vi "Write Page Properties.vi"(8 "error in (no error)":errorcluster, 10 "Page Properties":T1[](array[typedef]), 11 "CustomDeviceRepo in":refnum<class "CustomDeviceRepo.lvclass">) -> (0 "error out":errorcluster, 3 "CustomDeviceRepo out":refnum<class "CustomDeviceRepo.lvclass">)   [LabVIEW 2014, in "CustomDeviceRepo.lvclass"]
uses:
  CustomDeviceRepo.lvclass
  Custom Device Type Defs/Page Properties.ctl
  Custom Device XML/Custom Device XML/Path Cluster.ctl
  Custom Device XML/Custom Device XML/help.ctl
  CustomDeviceRepo.lvclass/CustomDeviceRepo.ctl
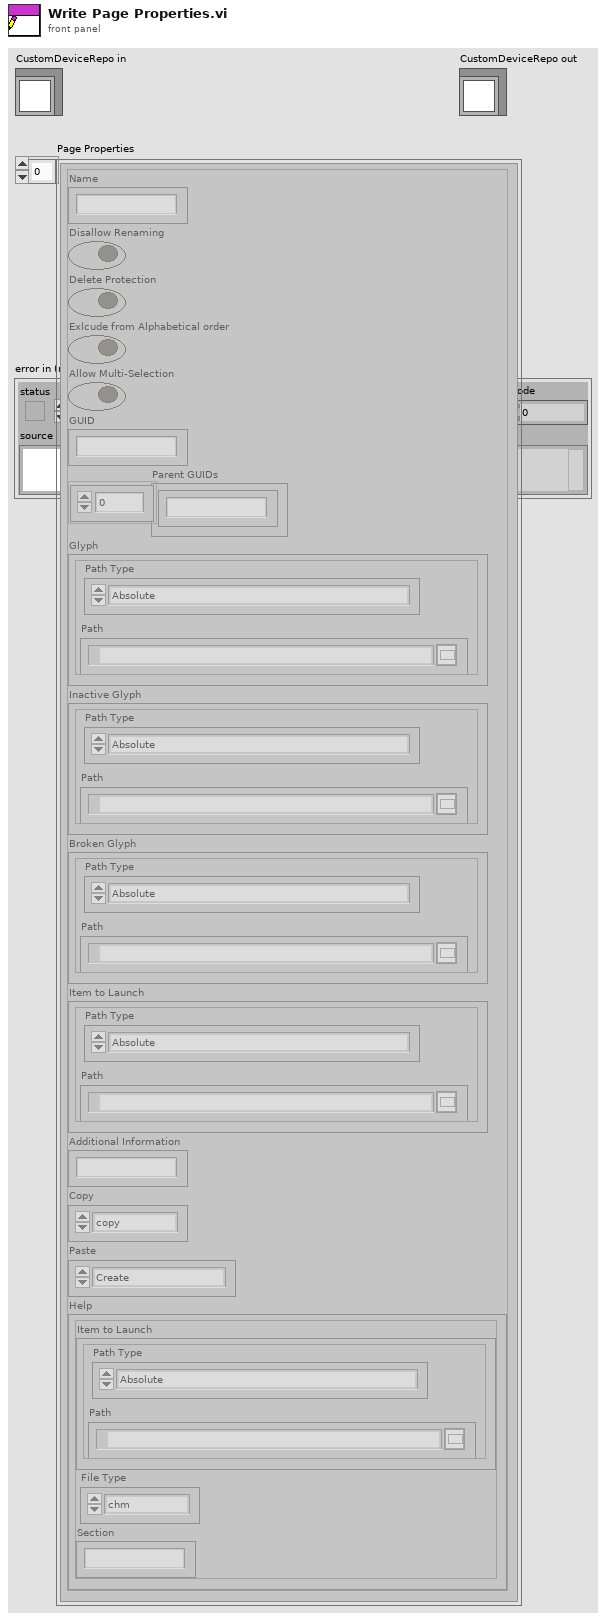
[diagram p1: front panel]
types:
  T1 = typedef "Page Properties.ctl" = cluster{"Name":string, "Disallow Renaming":bool, "Delete Protection":bool, "Exlcude from Alphabetical order":bool, "Allow Multi-Selection":bool, "GUID":string, "Parent GUIDs":string[], "Glyph":T2, "Inactive Glyph":T2, "Broken Glyph":T2, "Item to Launch":T2, "Additional Information":string, "Copy":enum16{"copy", "disabled"}, "Paste":enum16{"Create", "CreatIfNotExists_GUID", "CreatIfNotExists_Name", "Replace", "Dialog"}, "Help":T3}
  T2 = typedef "Path Cluster.ctl" = cluster{"Path":path, "Path Type":enum16{"Absolute", "To Base", "To Common Doc Dir", "To Application Data Dir"}}
  T3 = typedef "help.ctl" = cluster{"Item to Launch":T2, "Section":string, "File Type":enum16{"chm", "other"}}
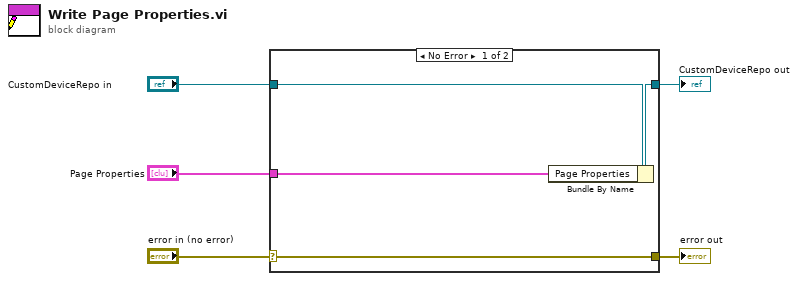
[diagram p0: block diagram]
diagram:
  n1 = case shown="No Error" "error in (no error)" {
    selector: "error in (no error)" -> [w9 w10]
    tunnel: [w9 w10] -> w4
    tunnel: [w7 w11] -> w2
    tunnel: "CustomDeviceRepo in" -> [w8 w11]
    tunnel: "Page Properties" -> [w6 _]
    frame No Error {
      n2 = Bundle By Name(cluster=w8, "Page Properties"=w6) -> (w7:refnum<class "CustomDeviceRepo.lvclass">)
    }
    frame Error {
    }
  }
  "error out" <- w4
  "CustomDeviceRepo out" <- w2
